vi "Create CT.vi"(8 "error in (no error)":errorcluster, 11 "Rocom Tests in":refnum<class "Rocom Tests.lvclass">) -> (0 "error out":errorcluster, 2 "Test Radio":refnum<class "SC Manufacturing Test.lvclass">, 3 "Rocom Tests out":refnum<class "Rocom Tests.lvclass">)   [LabVIEW 2015, in "Rocom Tests.lvclass"]
uses:
  Rocom Tests.lvclass
  Classes/Manufacturing Test/Class/SC Manufacturing Test.lvclass
  <vilib>/Cree, Inc/Cree Test Framework/Classes/Base Objects/Base Class/Base Class/Base Class.lvclass
  Test Class/Test Class.lvclass
  Classes/Application/Class/Application.lvclass
  Classes/Test Recipe/Class/Test Recipe.lvclass
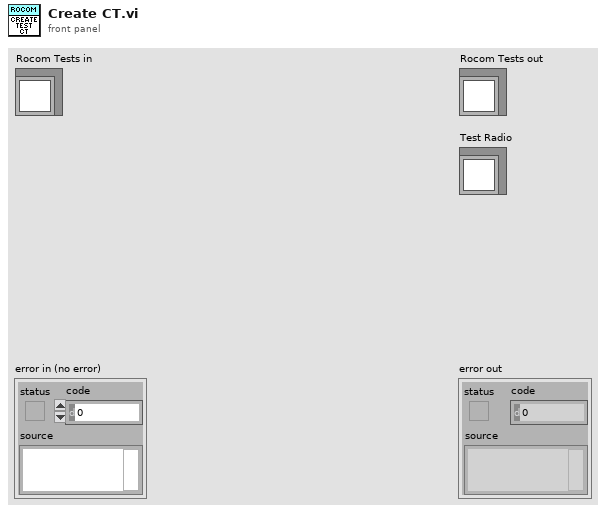
[diagram p1: front panel]
types:
  T1 = typedef "Application.lvlib/App Properties.lvclass/Class Properties -- Cluster.ctl" = cluster{"UUT Info":T2[], "Test Information":refnum<vi>, "Test Complete Event":refnum<user-event>, "Shop Floor System":refnum<class "Shop Floor System.lvclass">, "Gold Board":refnum<class "Golden Board.lvclass">, "Test Recipe":refnum<class "Test Recipe.lvclass">, "Instruments":refnum<class "Instrument.lvclass">[], "Mode":T3, "Test Results":cluster{"Pass":bool[], "Fail Codes":string[]}, "Station Config":refnum<class "Station Config.lvclass">}
  T2 = typedef "Application.lvlib/App Properties.lvclass/UUT Reference -- Cluster.ctl" = cluster{"Serial Number Reference":refnum<vi>, "Status Message Reference":refnum<vi>}
  T3 = typedef "Application.lvlib/Application.lvclass/Op Mode -- Enum.ctl" = u16
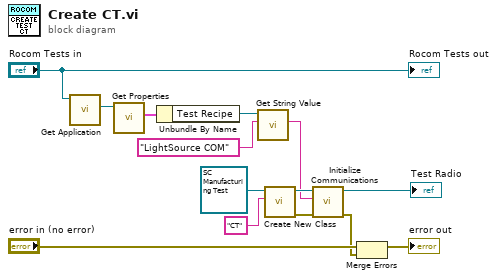
[diagram p0: block diagram]
diagram:
  n1 = call "Get Application.vi"("Test Class in"="Rocom Tests in") -> ("Application.lvlib:Application.lvclass"=w10:refnum<class "Application.lvclass">)  [unwired: 9 in, 1 out]
  n2 = call "Get Properties.vi"("Acrobat Template in"=w10) -> ("Class Properties"=w8:T1)  [unwired: 8 in, 2 out]
  n3 = Unbundle By Name(w8) -> ("Test Recipe"=w7:refnum<class "Test Recipe.lvclass">)
  n4 = call "Get String Value.vi"("Name"="LightSource COM", "Test Recipe in"=w7) -> ("Value"=w5:string)  [unwired: 7 in, 2 out]
  n5 = call <vilib>:"Create New Class.vi"("Name"="CT", "Base Class in"=refnum<class "SC Manufacturing Test.lvclass"> refnum ("SC Manufacturing Test.lvlib:SC Manufacturing Test.lvclass")) -> ("error out"=w4:errorcluster, "Base Class out"=w11:refnum<class "SC Manufacturing Test.lvclass">)  [unwired: 8 in]
  n6 = call "Initialize Communications.vi"("error in (no error)"=w4, "COM Port"=w5, "Acrobat Template in"=w11) -> ("error out"=w2:errorcluster, "Acrobat Template out"=→"Test Radio":refnum<class "SC Manufacturing Test.lvclass">)  [unwired: 7 in]
  n7 = Merge Errors("error in (no error)", w2) -> (→"error out":errorcluster)
  "Rocom Tests out" <- "Rocom Tests in"
